vi "rotate_point_by_radians_double.vi"(9 "theta":dbl, 10 "y":dbl, 11 "x":dbl) -> (2 "y out":dbl, 3 "x out":dbl)   [LabVIEW 2019]
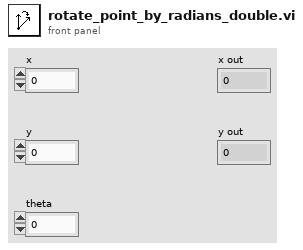
[diagram p1: front panel]
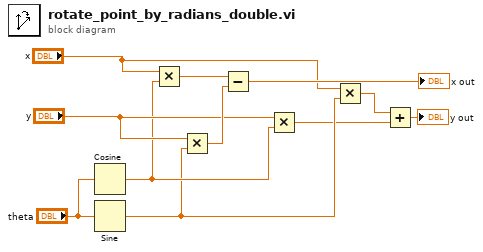
[diagram p0: block diagram]
diagram:
  n1 = Cosine(x="theta") -> (cos(x)=w7:dbl)
  n2 = Sine(x="theta") -> (sin(x)=w5:dbl)
  n3 = Multiply(x="x", y=w7) -> (x*y=w10:dbl)
  n4 = Multiply(x="y", y=w5) -> (x*y=w9:dbl)
  n5 = Subtract(x=w10, y=w9) -> (x-y=→"x out":dbl)
  n6 = Multiply(x="y", y=w7) -> (x*y=w3:dbl)
  n7 = Multiply(x="x", y=w5) -> (x*y=w4:dbl)
  n8 = Add(x=w4, y=w3) -> (x+y=→"y out":dbl)
